vi "Koheras_Communication.vi"(3 "Error in":errorcluster, 4 "Answer length":u32, 5 "Command":string, 6 "VISA resource name in":refnum<visa-resource-name>) -> (0 "Error out":errorcluster, 1 "Returns":string, 2 "VISA resource name out":refnum<visa-resource-name>)   [LabVIEW 2011]
uses:
  <vilib>/Utility/error.llb/DialogType.ctl
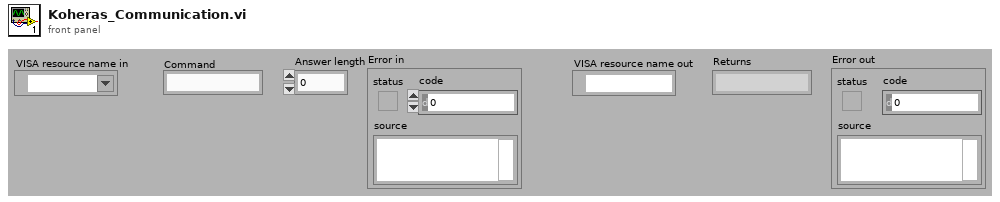
[diagram p1: front panel]
types:
  T1 = typedef "DialogType.ctl" = u16
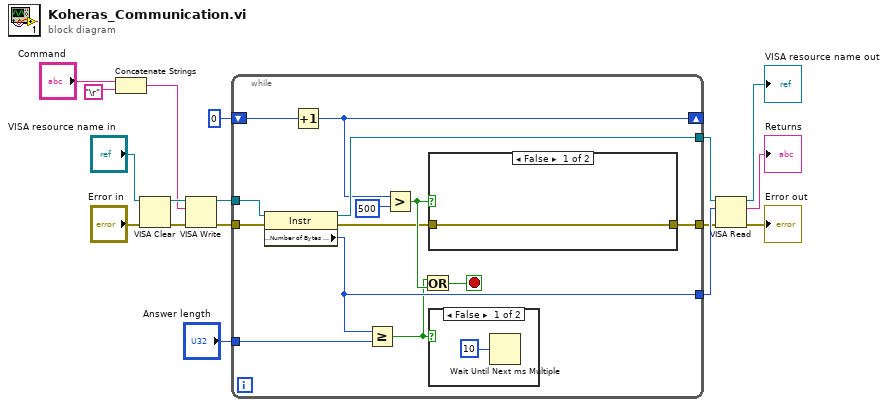
[diagram p0: block diagram]
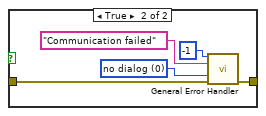
[diagram p3: hidden frame]
diagram:
  n1 = Concatenate Strings("Command", "\r") -> (w6:string)
  n2 = VISA Clear(VISA resource name="VISA resource name in", error in (no error)="Error in") -> (VISA resource name out=w9:refnum<visa-resource-name>, error out=w8:errorcluster)
  n3 = VISA Write(VISA resource name=w9, write buffer=w6, error in (no error)=w8) -> (VISA resource name out=w10:refnum<visa-resource-name>, error out=w11:errorcluster)  [unwired: 1 out]
  n4 = while {
    tunnel: w10 -> [w30]
    tunnel: w11 -> [w29]
    tunnel: [w19] -> w12
    tunnel: [w28] -> w13
    tunnel: [w27] -> w14
    tunnel: "Answer length" -> [w26]
    shift-right: [w23] -> _
    shift-left: u32 0 ("Answer length") -> [w25]
    stop <- w24 stop-if-true
    n5 = property class="Instr"(reference=w30, error in=w29) -> (reference out=w28:refnum<visa-resource-name>, error out=w20:errorcluster, "Serial Settings:Number of Bytes at Serial Port"=w27:u32)
    n6 = Increment(x=w25) -> (x+1=w23:u32)
    n7 = Greater Or Equal?(x=w27, y=w26) -> (x >= y?=w18:bool)
    n8 = Greater?(x=w23, y=u32 500) -> (0:w21:bool)
    n9 = Or(x=w18, y=w21) -> (x .or. y?=w24:bool)
    n10 = case shown="False" w21 {
      tunnel: w20 -> [w32 w37]
      tunnel: [w32 w36] -> w19
      frame False {
      }
      frame True {
        w35 = T1 0 items=["no dialog", "OK message", "continue or stop message", "OK message + warnings", "continue/stop + warnings"] ("type of dialog (OK msg:1)")
        n11 = call <vilib>:"General Error Handler.vi"("[error code] (0)"=-1, "[error source] (\" \")"="Communication failed" ("[error source] (\" \")"), "type of dialog (OK msg:1)"=w35, "error in (no error)"=w37) -> ("error out"=w36:errorcluster)  [unwired: 7 in, 4 out]
      }
    }
    n12 = case shown="False" w18 {
      frame False {
        n13 = Wait Until Next ms Multiple(millisecond multiple=u32 10) -> ()  [unwired: 1 out]
      }
      frame True {
      }
    }
  }
  n14 = VISA Read(VISA resource name=w13, byte count=w14, error in (no error)=w12) -> (VISA resource name out=→"VISA resource name out":refnum<visa-resource-name>, read buffer=→"Returns":string, error out=→"Error out":errorcluster)  [unwired: 1 out]
